vi "NanotecSMCPD.initialize.vi"(0 "i ref in":refnum<vi>, 1 "queryID":bool, 2 "resetControllers":bool, 3 "ms timeout (10000)":i32=10000, 5 "error in (no error)":errorcluster) -> (14 "i ref out":refnum<vi>, 15 "deviceID":string, 17 "timed out":bool, 19 "error out":errorcluster)   [LabVIEW 2014, in "NanotecSMCPD.lvlib"]
doc: "Initializes the instrument driver, reads the axes IDs and possibly resets all axes."
uses:
  NanotecSMCPD.lvlib
  CS_Core/CSSystem/CoreDefs/CoreDefs.error_type.ctl
  CS_Core/CSSystem/CoreDefs/CoreDefs.error_severity.ctl
  CS_Core/CSApplicationBaseClasses/MotorBase/MotorBase.lvlib
  CS_Core/CSSystem/CoreLib/CoreLib.lvlib
  instr.lib/NanotecSMCPD/NanotecSMCPDDriver.lvlib
  CSlibraries/UtilityLib/UtilityLib.lvlib
  CS_Core/CSApplicationBaseClasses/DeviceBase/DeviceBase.lvlib
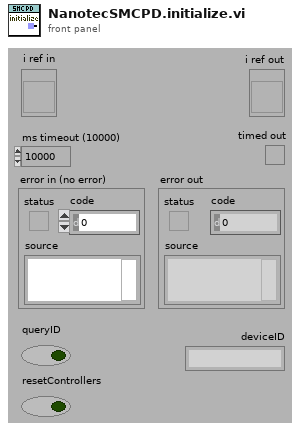
[diagram p1: front panel]
types:
  T1 = typedef "CoreDefs.error_severity.ctl" = enum16{"undefined", "information", "warning", "error", "fatal"}
  T2 = typedef "CoreDefs.error_type.ctl" = enum16{"no error", "can't load process", "can't unload process", "process does not exist", "can't install process", "can't remove process", "unknown function", "time out", "can't execute function", "duplicate queue name", "super not found", "caller queue invalid", "can't ping process", "unknown error", "VISA Error", "VISA timeout", "GPIB timeout", "GPIB error", "communication error", "data type mismatch", "can't read data from OPC server", "can't write data to OPC server", "OET error", "function not implemented", "process already exists", "invalid Shared Variable name", "error writing Shared Variable", "error reading Shared Variable", "invalid client name", "corrupt database", "unknown class", "call not authorized", "parameter out of range", "OET timeout: can't get data to modify", "invalid queue name", "requested operation incompatible with current state", "event undefined", "event disabled", "state undefined", "caller is not a friend", "EventBuilder: bad eventID", "EventBuilder: no DAQ devices", "a thread must not stop itself", "UNUSED ELEMENT4", "DiscArchiver: eventData incomplete", "DiscArchiver: eventData does not belong to run", "DiscArchiver: can't open file", "DiscArchiver: can't write to file", "DiscArchiver: available disc space low", "can't acquire semaphore", "error reading data from database", "notifier object is not existing", "can't register process", "can't unregister process", "illegal event type", "object disabled", "object already exists", "can't change state", "Instrument not found", "no connection to remote node", "invalid reference", "N/A", "UNUSED ELEMENT 1", "element not found", "illegal TCP/IP connection detected", "object does not exist", "invalid access ID", "unknown CS system", "invalid privilige", "unsupported data type", "unsupported server type", "IO server already exists", "Shared Variable already exists"}
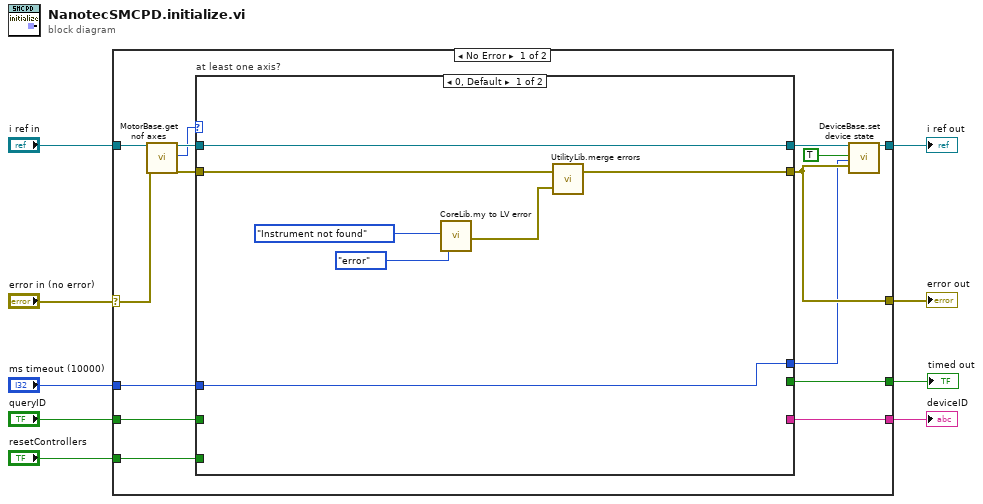
[diagram p0: block diagram]
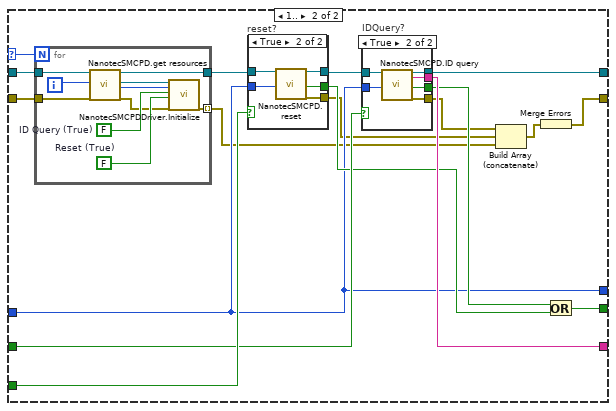
[diagram p2: hidden frame]
diagram:
  n1 = case shown="No Error" "error in (no error)" {
    selector: "error in (no error)" -> [w22 w73]
    tunnel: "i ref in" -> [w24 w74]
    tunnel: [w12 w74] -> w8
    tunnel: [w13 w73] -> w7
    tunnel: "ms timeout (10000)" -> [w21 _]
    tunnel: "queryID" -> [w18 _]
    tunnel: "resetControllers" -> [w17 _]
    tunnel: [w16 _] -> w2
    tunnel: [w15 _] -> w1
    frame No Error {
      n2 = call "MotorBase.get nof axes.vi"("i ref in"=w24, "error in (no error)"=w22) -> ("i ref out"=w23:refnum<vi>, "nOfAxis"=w19:i32, "error out"=w20:errorcluster)  [unwired: 15 in]
      n3 = case "at least one axis?" shown="0, Default" w19 {
        selector: w19 -> [_ w37]
        tunnel: w23 -> [w31 w44]
        tunnel: w21 -> [w25 w38]
        tunnel: w20 -> [w28 w43]
        tunnel: [w31 w45] -> w14
        tunnel: [w26 w32] -> w13
        tunnel: w18 -> [_ w48]
        tunnel: w17 -> [_ w49]
        tunnel: [_ w41] -> w16
        tunnel: [_ w47] -> w15
        tunnel: [w25 w38] -> w11
        frame 0, Default {
          n4 = call "CoreLib.my to LV error.vi"("ErrorTypes"=CoreDefs.error_type."Instrument not found", "severityLevel"=CoreDefs.error_severity."error") -> ("myErrorCluster"=w27:errorcluster)  [unwired: 16 in, 1 out]
          n5 = call "UtilityLib.merge errors.vi"("error2 (no error)"=w27, "error1 (no error)"=w28) -> ("error out"=w26:errorcluster)
        }
        frame 1.. {
          n6 = for {
            N: w37 -> [_]
            tunnel: w44 -> [w59]
            tunnel: w43 -> [w58]
            tunnel: [w52] -> w42
            tunnel: [w51] -> w34 mode=indexing
            i -> [w50]
            w54 = FALSE  # Reset (True)
            w55 = FALSE  # ID Query (True)
            n7 = call "NanotecSMCPD.get resources.vi"("i ref in"=w59, "axisNumber"=w50, "error in (no error)"=w58) -> ("i ref out"=w52:refnum<vi>, "VISA resource"=w57:refnum<visa-resource-name>, "address"=w56:i32, "error out"=w53:errorcluster)  [unwired: 13 in]
            n8 = call "NanotecSMCPDDriver.Initialize.vi"("VISA resource name"=w57, "contollerID"=w56, "ID Query (True)"=w55, "Reset (True)"=w54, "error in (no error)"=w53) -> ("error out"=w51:errorcluster)  [unwired: 12 in, 2 out]
          }
          n9 = case "reset?" shown="True" w49 {
            tunnel: w42 -> [w60 w65]
            tunnel: w38 -> [_ w64]
            tunnel: [w60 w63] -> w46
            tunnel: [_ w62] -> w35
            tunnel: [_ w61] -> w39
            frame False {
            }
            frame True {
              n10 = call "NanotecSMCPD.reset.vi"("i ref in"=w65, "ms timeout (10000)"=w64) -> ("i ref out"=w63:refnum<vi>, "timed out"=w61:bool, "error out"=w62:errorcluster)  [unwired: 15 in]
            }
          }
          n11 = case "IDQuery?" shown="True" w48 {
            tunnel: w46 -> [w66 w72]
            tunnel: w38 -> [_ w71]
            tunnel: [w66 w70] -> w45
            tunnel: [_ w69] -> w36
            tunnel: [_ w68] -> w47
            tunnel: [_ w67] -> w40
            frame False {
            }
            frame True {
              n12 = call "NanotecSMCPD.ID query.vi"("i ref in"=w72, "ms timeout (10000)"=w71) -> ("i ref out"=w70:refnum<vi>, "deviceID"=w68:string, "timed out"=w67:bool, "error out"=w69:errorcluster)  [unwired: 14 in]
            }
          }
          n13 = Build Array (concatenate)(w36, w35, w34) -> (w33:errorcluster[])
          n14 = Merge Errors(w33) -> (w32:errorcluster)
          n15 = Or(x=w40, y=w39) -> (x .or. y?=w41:bool)
        }
      }
      n16 = call "DeviceBase.set device state.vi"("i ref in"=w14, "implicit"=TRUE, "ms timeout (10000)"=w11, "device error"=w13) -> ("i ref out"=w12:refnum<vi>)  [unwired: 13 in, 2 out]
    }
    frame Error {
    }
  }
  "error out" <- w7
  "i ref out" <- w8
  "timed out" <- w2
  "deviceID" <- w1
